vi "convertToKeyValuePair_1Ddouble.vi"(8 "error in (no error)":errorcluster, 9 "presicion (0)":u8, 10 "value":dbl[](array[numeric]), 11 "name":string) -> (0 "error out":errorcluster, 3 "string converted":string)   [LabVIEW 2018]
doc: "Convert a 1-dimension double array into a key value pair as string."
uses:
  convertToKeyValuePair_string.vi
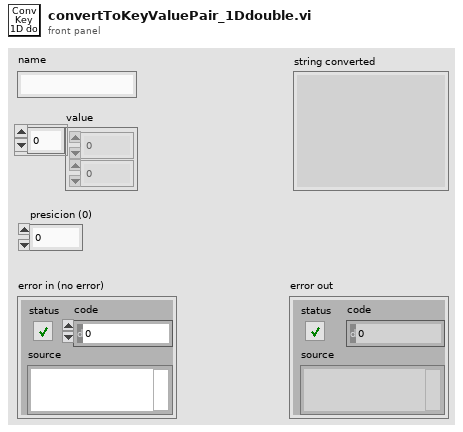
[diagram p1: front panel]
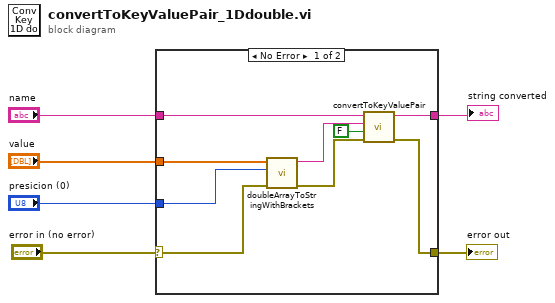
[diagram p0: block diagram]
diagram:
  n1 = case shown="No Error" "error in (no error)" {
    selector: "error in (no error)" -> [w9 w16]
    tunnel: "value" -> [w12 _]
    tunnel: "name" -> [w14 _]
    tunnel: "presicion (0)" -> [w11 _]
    tunnel: [w13 w16] -> w2
    tunnel: [w15 _] -> w1
    frame No Error {
      n2 = call "doubleArrayToStringWithBrackets.vi"("error in (no error)"=w9, "presicion (0)"=w11, "value"=w12) -> ("error out"=w8:errorcluster, "String"=w10:string)  [unwired: 7 in]
      n3 = call-poly "convertToKeyValuePair.vi"("error in (no error)"=w8, "double quotes (T)"=FALSE ("double quotes (F)"), "value"=w10, "name"=w14) -> ("error out"=w13:errorcluster, "string converted"=w15:string)  [unwired: 6 in]
    }
    frame Error {
    }
  }
  "error out" <- w2
  "string converted" <- w1
